vi "test BNR and BCD Parameters that Span Words.vi"(8 "error in":errorcluster, 11 "Loopback in":refnum<class "Loopback.lvclass">) -> (0 "error out":errorcluster, 3 "Loopback out":refnum<class "Loopback.lvclass">)   [LabVIEW 2020, in "Loopback.lvclass"]
uses:
  Loopback.lvclass
  C:/Users/nitest/Desktop/Git 2020/niveristand-custom-device-testing-tools/VeriStandTestCase/VeriStandTestCase.lvclass
  niveristand-custom-device-testing-tools/VeriStandTestUtilities/VeriStandTestUtilities.lvlib
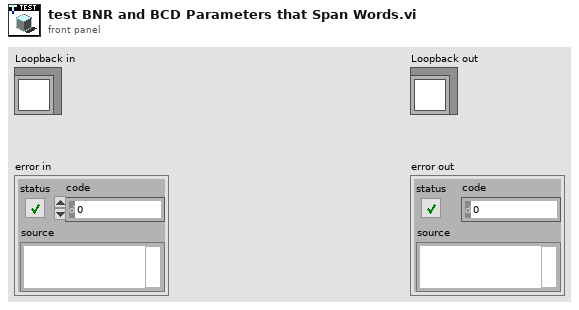
[diagram p1: front panel]
types:
  T1 = typedef "NI_VS Workspace ExecutionAPI.lvlib/WorkspaceAPI.ctl" = refnum<k24>
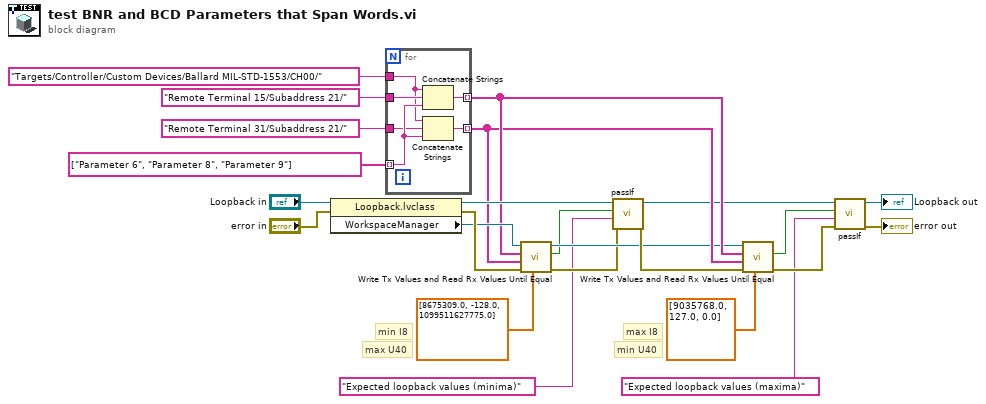
[diagram p0: block diagram]
diagram:
  # "min U40"
  # "max I8"
  # "min I8"
  # "max U40"
  n1 = property class="Loopback.lvclass"(reference="Loopback in", error in="error in") -> (reference out=w21:refnum<class "Loopback.lvclass">, error out=w22:errorcluster, "WorkspaceManager"=w20:T1)
  n2 = for {
    tunnel: "Remote Terminal 15/Subaddress 21/" ("Channel") -> [w29]
    tunnel: string[] ["Parameter 6", "Parameter 8", "Parameter 9"] ("Channels") -> [w28] mode=indexing
    tunnel: [w30] -> w16 mode=indexing
    tunnel: "Remote Terminal 31/Subaddress 21/" ("Channel") -> [w27]
    tunnel: [w26] -> w15 mode=indexing
    tunnel: "Targets/Controller/Custom Devices/Ballard MIL-STD-1553/CH00/" ("base name for channel aliases") -> [w25]
    n3 = Concatenate Strings(w25, w29, w28) -> (w30:string)
    n4 = Concatenate Strings(w25, w27, w28) -> (w26:string)
  }
  n5 = call "Write Tx Values and Read Rx Values Until Equal.vi"("Tx values"=dbl[] [8675309.0, -128.0, 1099511627775.0] ("appended array"), "error in"=w22, "Rx aliases"=w15, "Tx aliases"=w16, "workspace manager in"=w20) -> ("error out"=w9:errorcluster, "values equal"=w10:bool, "workspace manager out"=w13:T1)  [unwired: 4 in]
  n6 = call-dynamic "passIf.vi"("error in (no error)"=w9, "message (\"\")"="Expected loopback values (minima)" ("message (\"\")"), "pass"=w10, "TestCase in"=w21) -> ("error out"=w14:errorcluster, "TestCase out"=w6:refnum<class "Loopback.lvclass">)  [unwired: 6 in]
  n7 = call "Write Tx Values and Read Rx Values Until Equal.vi"("Tx values"=dbl[] [9035768.0, 127.0, 0.0] ("appended array"), "error in"=w14, "Rx aliases"=w15, "Tx aliases"=w16, "workspace manager in"=w13) -> ("error out"=w17:errorcluster, "values equal"=w18:bool)  [unwired: 4 in, 1 out]
  n8 = call-dynamic "passIf.vi"("error in (no error)"=w17, "message (\"\")"="Expected loopback values (maxima)" ("message (\"\")"), "pass"=w18, "TestCase in"=w6) -> ("error out"=→"error out":errorcluster, "TestCase out"=→"Loopback out":refnum<class "Loopback.lvclass">)  [unwired: 6 in]
